vi "Format to string.vi"(8 "error in (no error)":errorcluster, 11 "address":refnum<class "Generic Network Address.lvclass">) -> (0 "error out":errorcluster, 2 "address string":string, 3 "address out":refnum<class "Generic Network Address.lvclass">)   [LabVIEW 2020, in "NI_WFCN.lvlib" / "Generic Network Address.lvclass"]
doc: "Returns a human-readable string representation of this address."
uses:
  <vilib>/net/WFCN/Addressing/Generic Network Address/Generic Network Address.lvclass
  <vilib>/net/WFCN/Addressing/Generic Network Address/Generic Network Address.lvclass/Generic Network Address.ctl
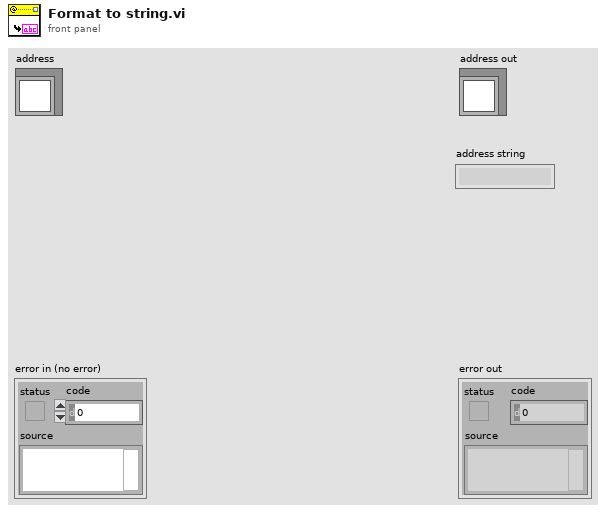
[diagram p1: front panel]
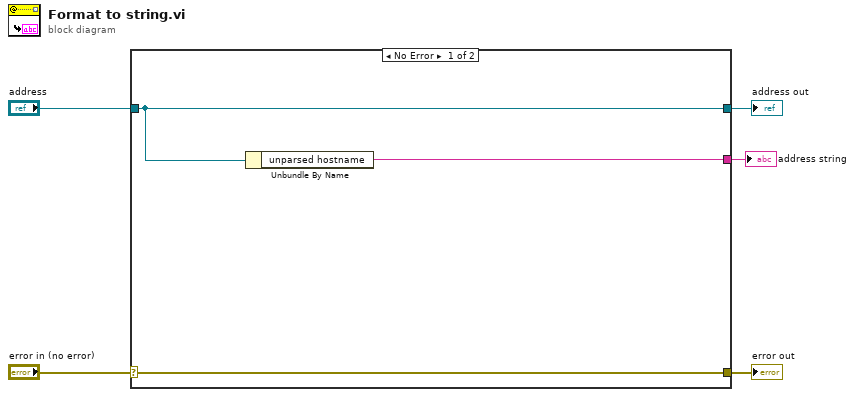
[diagram p0: block diagram]
diagram:
  n1 = case shown="No Error" "error in (no error)" {
    selector: "error in (no error)" -> [w8 w10]
    tunnel: [w8 w10] -> w4
    tunnel: [w7 w9] -> w2
    tunnel: "address" -> [w7 w9]
    tunnel: [w6 _] -> w1
    frame No Error {
      n2 = Unbundle By Name(w7) -> ("unparsed hostname"=w6:string)
    }
    frame Error {
    }
  }
  "error out" <- w4
  "address out" <- w2
  "address string" <- w1
